vi "锯齿波子vi.vi"(10 "幅值":dbl) -> (2 "数组":dbl[](array[numeric]))   [LabVIEW 2018]
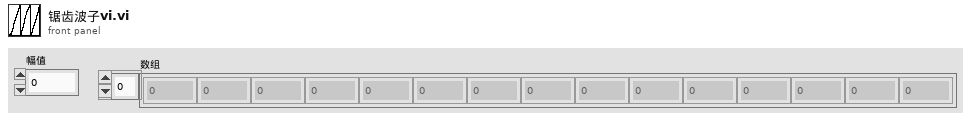
[diagram p1: front panel]
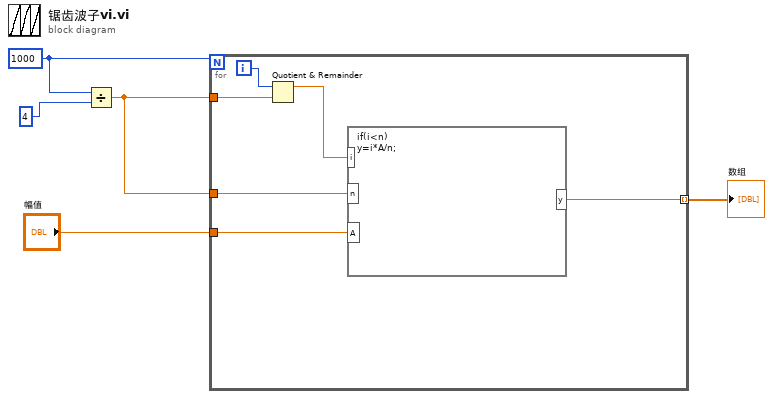
[diagram p0: block diagram]
diagram:
  w4 = 1000
  n1 = Divide(x=w4, y=4) -> (x/y=w3:dbl)
  n2 = for {
    N: w4 -> [_]
    tunnel: w3 -> [w10]
    tunnel: w3 -> [w8]
    tunnel: "幅值" -> [w7]
    tunnel: [w6] -> w1 mode=indexing
    i -> [w11]
    n3 = Quotient & Remainder(x=w11, y=w10) -> (x-y*floor(x/y)=w9:dbl)  [unwired: 1 out]
    n4 = formula code="if(i<n)\ny=i*A/n;"("i"=w9, "n"=w8, "A"=w7) -> ("y"=w6:dbl)
  }
  "数组" <- w1
